vi "initialisePPData.vi"   [LabVIEW 2017]
uses:
  Controls/postProData.ctl
  Controls/U.ctl
  Controls/blocksWTInfo.ctl
  Globals/measurementGlobal.vi
types:
  T1 = typedef "blocksWTInfo.ctl" = cluster{"Velocity (ms^-1)":dbl, "Density (kgm^-3)":dbl, "Pressure (Pa)":dbl, "Temperature (C)":dbl}
  T2 = typedef "U.ctl" = cluster{"Samples":dbl, "U":dbl, "U2":dbl, "U3":dbl, "U4":dbl}
  T3 = typedef "postProData.ctl" = cluster{"Channel":string, "Samples":i32, "U":dbl, "u^2":dbl, "u^3":dbl, "u^4":dbl, "Kurtosis":dbl, "Skewness":dbl, "Turb":dbl}
  T4 = typedef "chanType.ctl" = enum16{"Default", "Chell 64-Channel"}
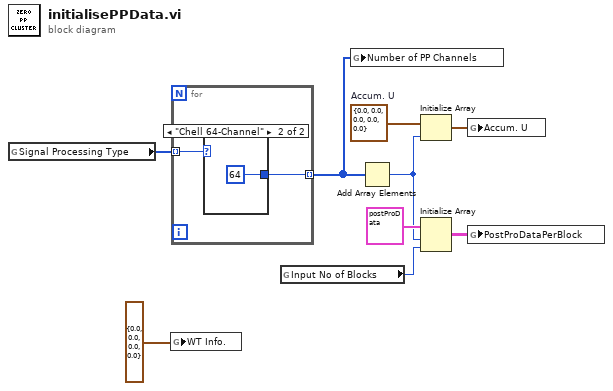
[diagram p0: block diagram]
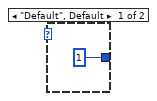
[diagram p2: hidden frame]
diagram:
  w5 = T2 {"Samples"=0.0, "U"=0.0, "U2"=0.0, "U3"=0.0, "U4"=0.0}  # Accum. U
  n1 = global read "measurementGlobal.vi" "Signal Processing Type"() -> (w9:T4[])
  n2 = global write "measurementGlobal.vi" "WT Info."(T1 {"Velocity (ms^-1)"=0.0, "Density (kgm^-3)"=0.0, "Pressure (Pa)"=0.0, "Temperature (C)"=0.0} ("WT Info.")) -> ()
  n3 = for {
    tunnel: w9 -> [w10] mode=indexing
    tunnel: [w11] -> w8 mode=indexing
    n4 = case shown="\"Chell 64-Channel\"" w10 {
      tunnel: [1 64] -> w11
      frame "Default", Default {
      }
      frame "Chell 64-Channel" {
      }
    }
  }
  n5 = global read "measurementGlobal.vi" "Input No of Blocks"() -> (w2:i32)
  n6 = global write "measurementGlobal.vi" "Number of PP Channels"(w8) -> ()
  n7 = Add Array Elements(numeric array=w8) -> (sum=w3:i32)
  n8 = Initialize Array(w5, w3) -> (w4:T2[])
  n9 = Initialize Array(T3 {"Channel"="", "Samples"=0, "U"=0.0, "u^2"=0.0, "u^3"=0.0, "u^4"=0.0, "Kurtosis"=0.0, "Skewness"=0.0, "Turb"=0.0} ("Post Pro Data"), w3, w2) -> (w6:T3[][])
  n10 = global write "measurementGlobal.vi" "Accum. U"(w4) -> ()
  n11 = global write "measurementGlobal.vi" "PostProDataPerBlock"(w6) -> ()
